vi "Links To.vi"(8 "error in (no error)":errorcluster, 10 "State Name":string, 11 "State in":refnum<class "State.lvclass">) -> (0 "error out":errorcluster, 1 "linked to?":bool, 3 "State out":refnum<class "State.lvclass">)   [LabVIEW 2015, in "State.lvclass"]
uses:
  State.lvclass
  State.lvclass/State.ctl
  Termination/Termination.lvclass/Termination.ctl
  Timeout/Timeout.lvclass/Timeout.ctl
  Termination/Read Link to.vi
  Timeout/Read Link to.vi
  Termination/Termination.lvclass
  Timeout/Timeout.lvclass
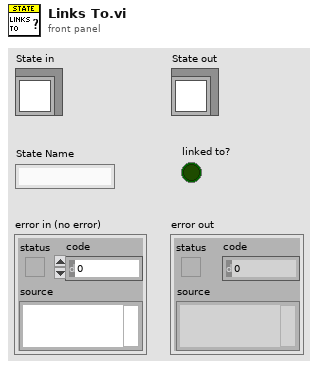
[diagram p1: front panel]
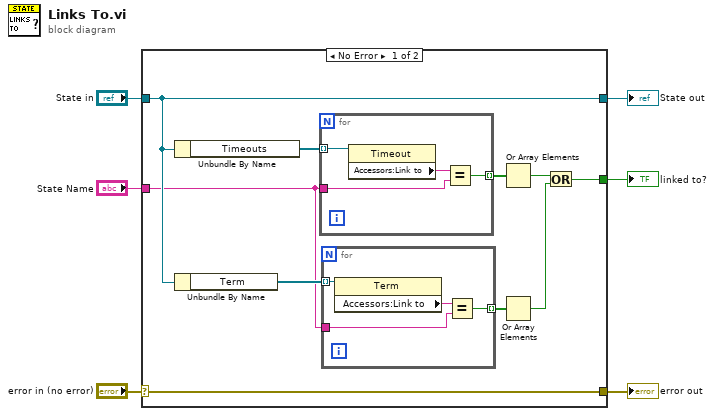
[diagram p0: block diagram]
diagram:
  n1 = case shown="No Error" "error in (no error)" {
    selector: "error in (no error)" -> [w16 w26]
    tunnel: [w16 w26] -> w5
    tunnel: [w14 w25] -> w3
    tunnel: "State in" -> [w14 w25]
    tunnel: "State Name" -> [w12 _]
    tunnel: [w7 _] -> w1
    frame No Error {
      n2 = Unbundle By Name(w14) -> ("Timeouts"=w15:refnum<class "Timeout.lvclass">[])
      n3 = Unbundle By Name(w14) -> ("Term"=w13:refnum<class "Termination.lvclass">[])
      n4 = for {
        tunnel: w15 -> [w24] mode=indexing
        tunnel: w12 -> [w22]
        tunnel: [w21] -> w11 mode=indexing
        n5 = property class="Timeout"(reference=w24) -> ("Accessors:Link to"=w23:string)  [unwired: 1 in, 2 out]
        n6 = Equal?(x=w23, y=w22) -> (x = y?=w21:bool)
      }
      n7 = for {
        tunnel: w13 -> [w20] mode=indexing
        tunnel: w12 -> [w18]
        tunnel: [w17] -> w10 mode=indexing
        n8 = property class="Term"(reference=w20) -> ("Accessors:Link to"=w19:string)  [unwired: 1 in, 2 out]
        n9 = Equal?(x=w19, y=w18) -> (x = y?=w17:bool)
      }
      n10 = Or Array Elements(Boolean array=w11) -> (logical OR=w9:bool)
      n11 = Or Array Elements(Boolean array=w10) -> (logical OR=w8:bool)
      n12 = Or(x=w9, y=w8) -> (x .or. y?=w7:bool)
    }
    frame Error {
    }
  }
  "error out" <- w5
  "State out" <- w3
  "linked to?" <- w1
